vi "Change File RW Attribute.vi"(8 "error in (no error)":errorcluster, 10 "Read/Write Attribute":enum16{"Read/Write", "Read Only"}(ring), 11 "Path Filter":string) -> (0 "error out":errorcluster)   [LabVIEW 2009]
doc: "Changes the read/write attribute of all files located in the <vilib>\\LapDog folder and subfolders where the file path includes the text defined by Path Filter."
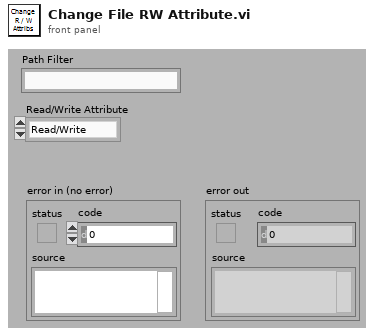
[diagram p1: front panel]
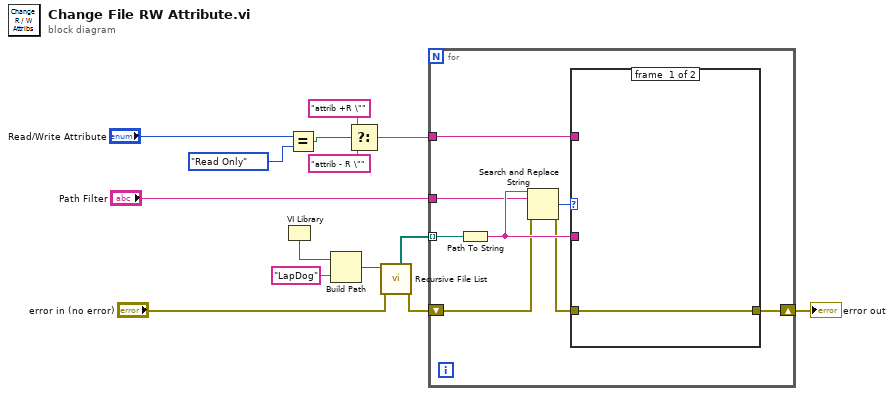
[diagram p0: block diagram]
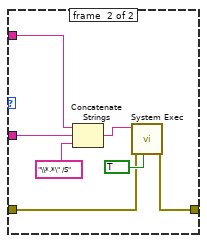
[diagram p2: hidden frame]
diagram:
  n1 = VI Library() -> (path=w13:path)
  n2 = Equal?(x="Read/Write Attribute", y=enum16{"Read/Write", "Read Only"}."Read Only" ("Read/Write Attribute")) -> (x = y?=w2:bool)
  n3 = Build Path(base path=w13, name or relative path="LapDog") -> (appended path=w11:path)
  n4 = Select(t="attrib +R \"" ("string"), s=w2, f="attrib - R \"" ("string")) -> (s? t:f=w1:string)
  n5 = call <vilib>:"Recursive File List.vi"("error in (no error)"="error in (no error)", "Folder Path"=w11) -> ("error out"=w8:errorcluster, "All Folders"=w14:path[])  [unwired: 5 in, 3 out]
  n6 = for {
    tunnel: w14 -> [w22] mode=indexing
    tunnel: "Path Filter" -> [w19]
    shift-right: [w16] -> w7
    shift-left: w8 -> [w18]
    tunnel: w1 -> [w15]
    n7 = Path To String(path=w22) -> (string=w20:string)
    n8 = Search and Replace String(input string=w20, search string=w19, error in=w18) -> (number of replacements=w21:i32, error out=w17:errorcluster)  [unwired: 5 in, 2 out]
    n9 = case shown="1.." w21 {
      tunnel: w20 -> [_ w30]
      tunnel: w17 -> [w23 w26]
      tunnel: [w23 w25] -> w16
      tunnel: w15 -> [_ w24]
      frame #0 {
      }
      frame #1 {
        n10 = Concatenate Strings(w24, w30, "\\*.*\" /S" ("string")) -> (w27:string)
        n11 = call <vilib>:"System Exec.vi"("run minimized? (F)"=TRUE, "error in (no error)"=w26, "command line"=w27) -> ("error out"=w25:errorcluster)  [unwired: 5 in, 3 out]
      }
    }
  }
  "error out" <- w7
